vi "Register for Events.vi"(8 "error in (no error)":errorcluster, 11 "XY Stage Controller in":refnum<class "XY Stage Controller.lvclass">) -> (0 "error out":errorcluster, 2 "Event Registration Refnum":refnum<event-registration>, 3 "XY Stage Controller out":refnum<class "XY Stage Controller.lvclass">)   [LabVIEW 2022 SP3, in "XY Stage Controller.lvclass"]
uses:
  XY Stage Controller.lvclass
  XY Stage Controller.lvclass/XY Stage Controller.ctl
  XY Stage Data Class/XY Stage Data Class.lvclass
  XY Stage Data Class/XY Position.ctl
  XY Stage Data Class/Moving.ctl
  XY Stage Data Class/Homed.ctl
  XY Stage Data Class/Acceleration.ctl
  XY Stage Data Class/Current Speed.ctl
  XY Stage Data Class/Events.ctl
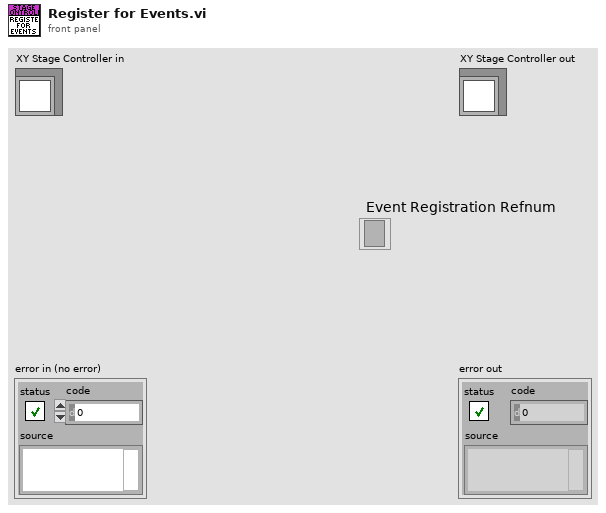
[diagram p1: front panel]
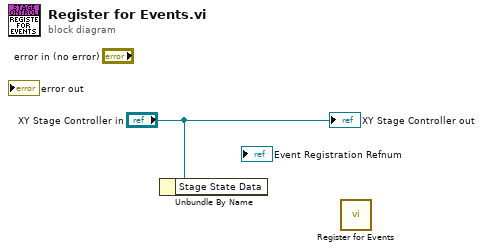
[diagram p0: block diagram]
diagram:
  n1 = Unbundle By Name("XY Stage Controller in") -> ()  [unwired: 1 out]
  n2 = call "Register for Events.vi"() -> ()  [unwired: 9 in, 3 out]
  "XY Stage Controller out" <- "XY Stage Controller in"
